vi "Process_data.vi"(0 "PWA Binary":i16[][](array[numeric]), 1 "Analogue Binary":i16[][](array[numeric]), 2 "LDA Binary output":u16[][](array[numeric]), 3 "Analogue volts":dbl[][](array[numeric]) format="%.2f", 4 "Measurement top level?":bool, 5 "Block Timings":T1={"Started"=0.0, "Ended"=0.0, "Analogue Frequency Hz"=1000.0} {"Analogue Frequency Hz" format="%.2f"}) -> (6 "Vel stat display":string[][](table), 7 "First Plot data":cluster{"Xo":dbl, "Delta X":dbl, dbl[]}[](array[cluster]) {"?" format="%.2f"; "Delta X" format="%.2f"; "Xo" format="%.2f"}, 8 "Second Plot data":cluster{"Xo":dbl, "Delta X":dbl, dbl[]}[](array[cluster]) {"?" format="%.2f"; "Delta X" format="%.2f"; "Xo" format="%.2f"}, 9 "Max Measurement time up":bool)   [LabVIEW 2010]
uses:
  Controls/Block_start_and_end.ctl
  Controls/Correlation_cluster.ctl
  Controls/Inst_type.ctl
  Controls/Instrument_Array.ctl
  Controls/Board_Types.ctl
  Globals/Meas_global.vi
  Globals/LDA_meas_global_1.vi
  Acquisition/PWA/PWAtasksGLOBAL.vi
  Globals/Dynamic_call_global.ph.vi
  Globals/Plug_in_data_global.vi
  <vilib>/Analysis/NI_AALBase.lvlib
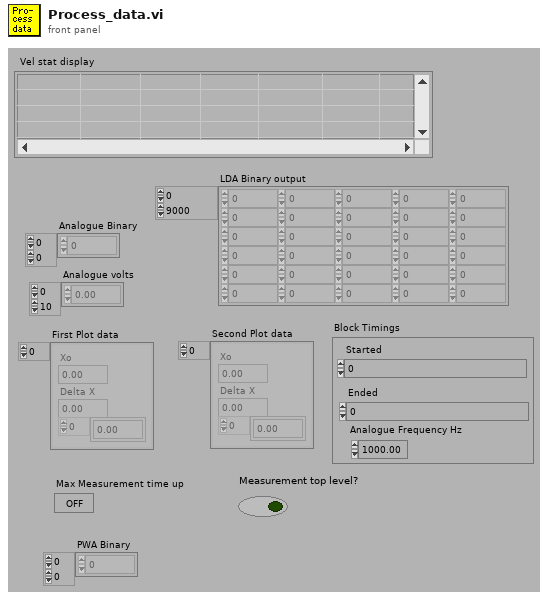
[diagram p1: front panel]
types:
  T1 = typedef "Block_start_and_end.ctl" = cluster{"Started":dbl, "Ended":dbl, "Analogue Frequency Hz":dbl}
  T2 = typedef "PWA_Data.ctl" = enum16{"No PWA Data", "One Ch PWA"}
  T3 = typedef "BSA_Type.ctl" = enum16{"57N11", "BSA F60"}
  T4 = typedef "Correlation_cluster.ctl" = cluster{"U inst":string, "W inst":string, "uw":dbl, "uw/u'w'":dbl, "u^2w":dbl, "uw^2":dbl, "uw^3":dbl, "u^3w":dbl, "u^2w^2":dbl}
  T5 = typedef "Inst_type.ctl" = enum16{"Propeller anemometer", "Raw voltage", "Pressure Transducer", "Pitot-static tube", "Preston tube", "Hot wire", "Cross wire 1", "Cross wire 2", "Generic Linear", "Generic Polynomial", "Generic BackPoly", "Fast FID", "Thermocouple", "Cold wire", "Pulsed Wire", "LDA Vel", "LDA Tran time", "LDA Arr time"}
  T6 = typedef "Instrument_Array.ctl" = enum16{"PWA", "LDA", "Analogue"}
  T7 = typedef "Board_Types.ctl" = enum16{"Simulate", "NB-MIO-16H", "PCI-MIO-16E", "6000E Series", "USB-92xx", "ADC488", "Lab-NB", "NB-DIO-24", "NI-DAQmx", "Local ADAM", "Server Channels"}
  T8 = typedef "Analysis_info_cluster.ctl" = cluster{"Colour":u32, "Inst type":T5, "Inst name":string, "Symbol":string, "Code name":string, "Extra Info":string, "Inst Array":T6, "Index":i32, "Voltage Index":i32, "Extra Titles":string[], "Extra Values":string[]}
  T9 = typedef "Post_Process.ctl" = enum16{"Take New Data", "Post Process Raw Data File"}
  T10 = typedef "Graph_Type.ctl" = enum16{"Show no graph", "Voltage trace", "Velocity trace", "Vel histogram", "Spectrum", "f.E(f) v Log f", "Auto-Corr"}
  T11 = cluster{"Plot 1":u16, "Plot 2":u16, "Save graph":u16, "Plot Type":T10}
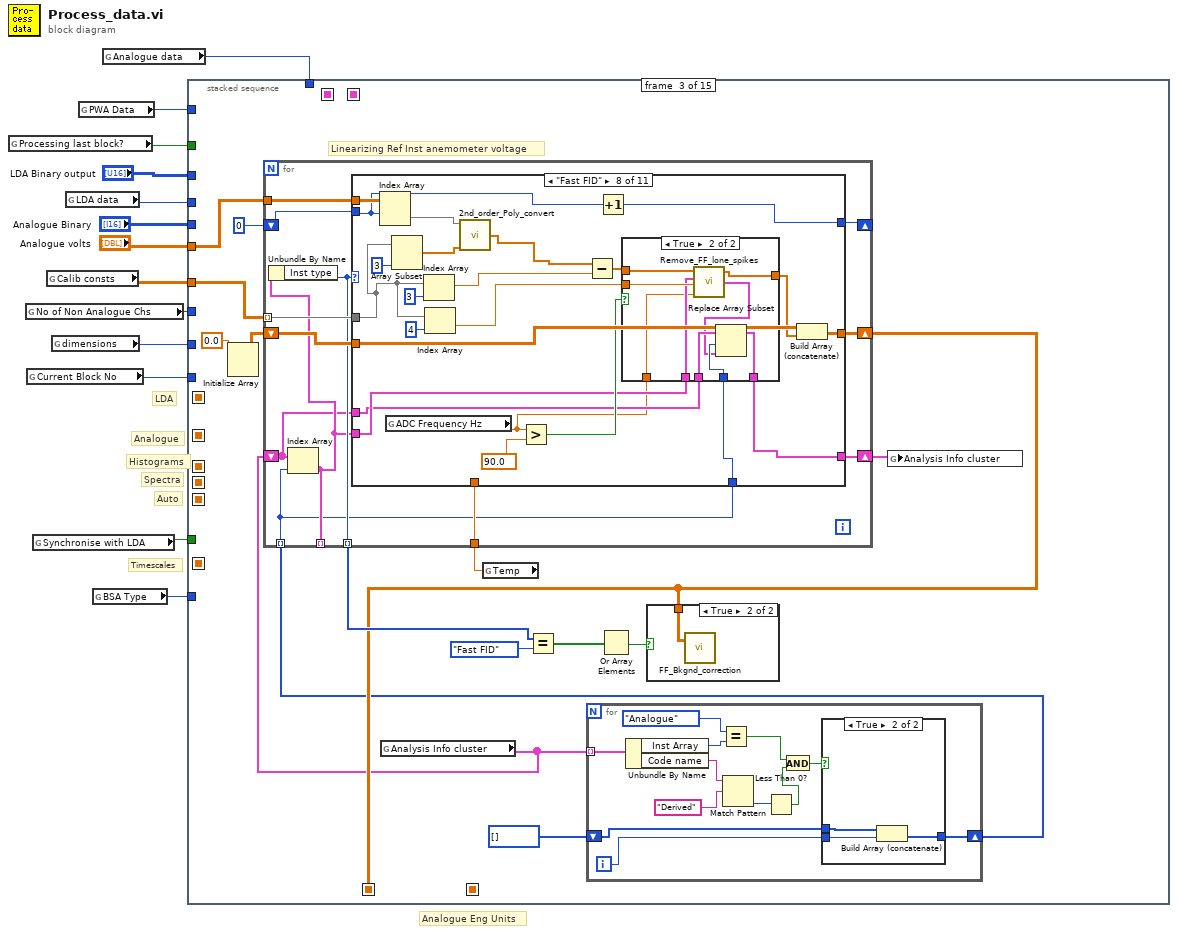
[diagram p0: block diagram]
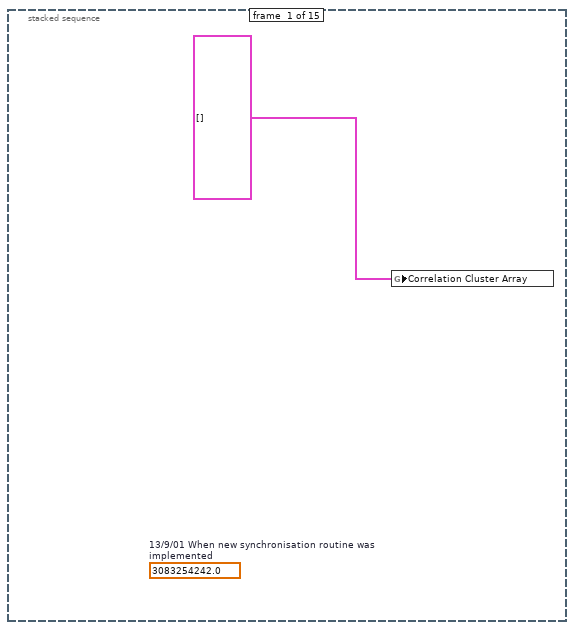
[diagram p2: hidden frame]
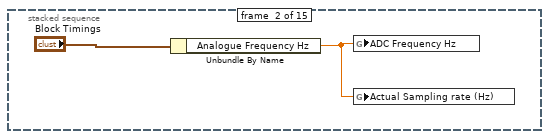
[diagram p3: hidden frame]
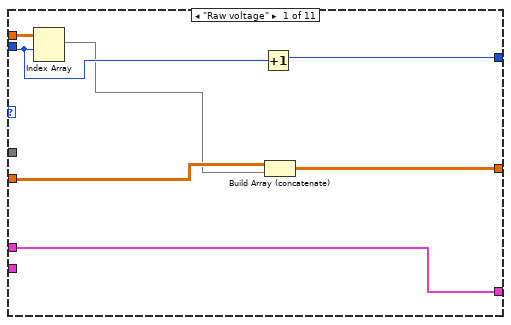
[diagram p6: hidden frame]
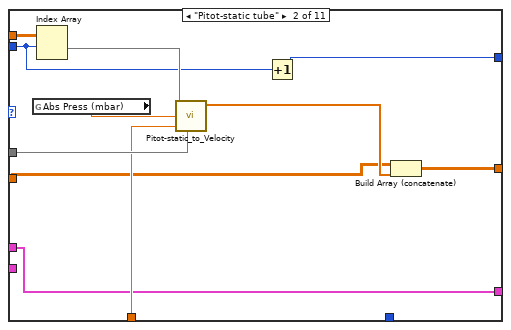
[diagram p7: hidden frame]
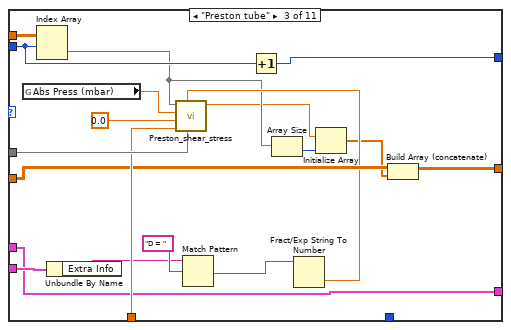
[diagram p8: hidden frame]
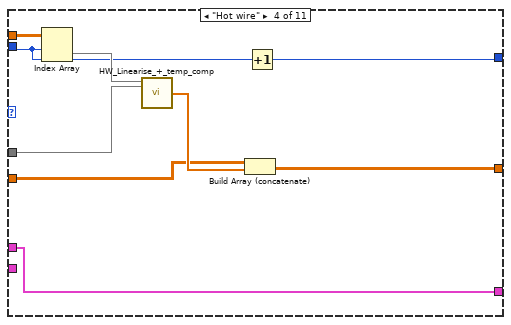
[diagram p9: hidden frame]
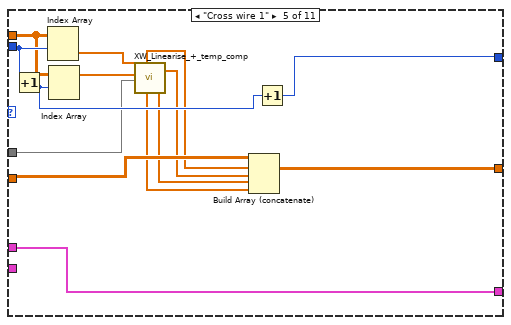
[diagram p10: hidden frame]
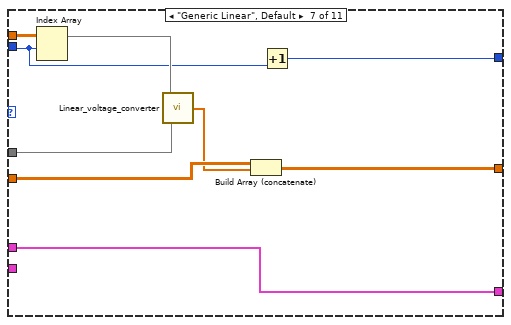
[diagram p12: hidden frame]
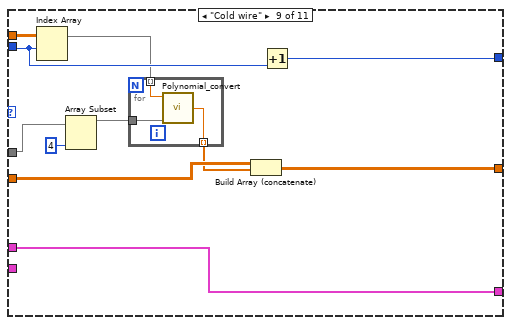
[diagram p14: hidden frame]
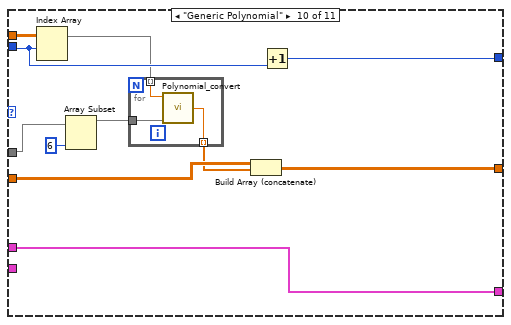
[diagram p15: hidden frame]
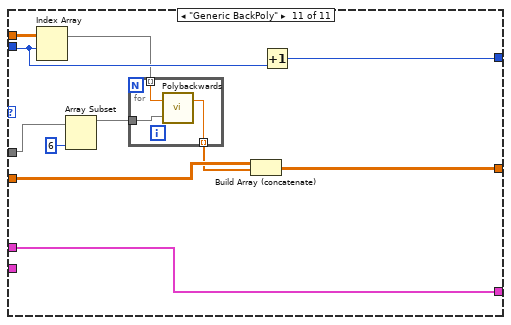
[diagram p16: hidden frame]
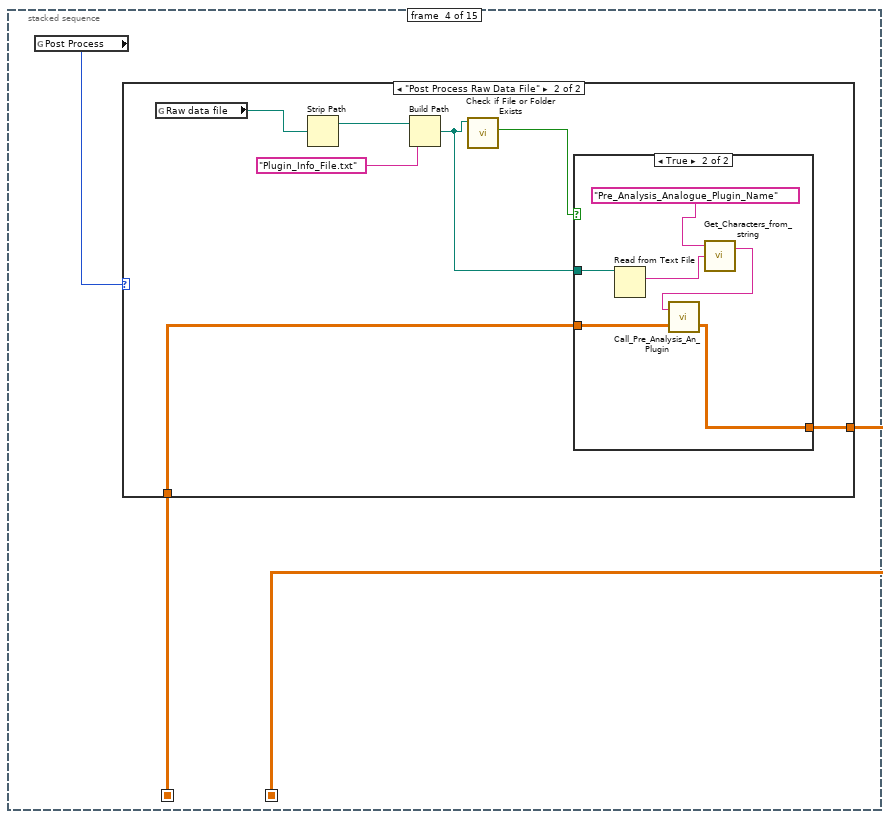
[diagram p17: hidden frame]
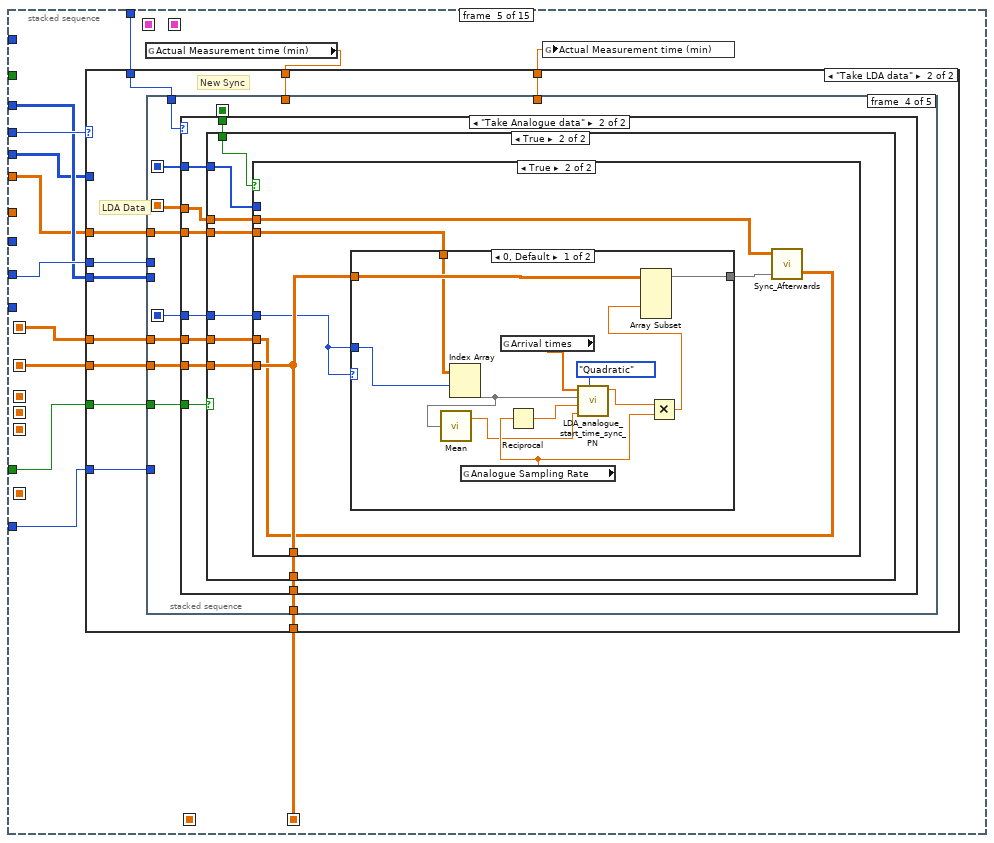
[diagram p20: hidden frame]
diagram:
  # "Timescales"
  # "LDA"
  # "Auto"
  # "Spectra"
  # "Histograms"
  # "Analogue Eng Units"
  # "Analogue"
  n1 = global read "Meas_global.vi" "Processing last block?"() -> (w9:bool)
  n2 = global read "Meas_global.vi" "No of Non Analogue Chs"() -> (w5:i32)
  n3 = global read "Meas_global.vi" "Current Block No"() -> (w10:i32)
  n4 = global read "Meas_global.vi" "Synchronise with LDA"() -> (w4:bool)
  n5 = global read "Meas_global.vi" "Calib consts"() -> (w3:dbl[][])
  n6 = global read "Meas_global.vi" "dimensions"() -> (w13:enum16{"1D", "2D"})
  n7 = global read "Meas_global.vi" "LDA data"() -> (w12:enum16{"No LDA data", "Take LDA data"})
  n8 = global read "Meas_global.vi" "PWA Data"() -> (w2:T2)
  n9 = global read "LDA_meas_global_1.vi" "BSA Type"() -> (w1:T3)
  n10 = global read "Meas_global.vi" "Analogue data"() -> (w11:enum16{"No Analogue data", "Take Analogue data"})
  n11 = stacked-sequence {
    seq-local: [_ _ _ _ w235 _ _ _ _ _ _ _ _ _ _] -> [_ _ _ _ _ _ w488 w501 w509 w524 w535 w554 w559 _ _]
    seq-local: [_ _ _ w210 _ _ _ _ _ _ _ _ _ _ _] -> [_ _ _ _ w237 _ _ _ _ _ _ _ _ _ _]
    seq-local: [_ _ _ _ _ _ w487 _ _ _ _ _ _ _ _] -> [_ _ _ _ _ _ _ _ _ w523 _ _ _ w602 _]
    seq-local: [_ _ _ _ _ _ _ w500 _ _ _ _ _ _ _] -> [_ _ _ _ _ _ _ _ _ w522 _ _ _ _ _]
    seq-local: [_ _ _ _ _ _ _ _ w508 _ _ _ _ _ _] -> [_ _ _ _ _ _ _ _ _ w521 w542 _ _ _ _]
    seq-local: [_ _ _ _ _ _ _ _ _ w516 _ _ _ _ _] -> [_ _ _ _ _ _ _ _ _ _ _ _ w565 _ _]
    seq-local: [_ _ _ _ _ _ _ _ _ w515 _ _ _ _ _] -> [_ _ _ _ _ _ _ _ _ _ _ _ w564 _ _]
    seq-local: [_ _ _ _ w232 _ _ _ _ _ _ _ _ _ _] -> [_ _ _ _ _ _ w489 _ _ w514 _ w555 w560 _ w611]
    seq-local: [_ _ _ _ _ _ _ _ _ _ w528 _ _ _ _] -> [_ _ _ _ _ _ _ _ _ _ _ w552 _ _ w610]
    seq-local: [_ _ w21 _ _ _ _ _ _ _ _ _ _ _ _] -> [_ _ _ w209 _ _ _ _ _ _ _ _ _ _ _]
    tunnel: w10 -> [_ _ _ _ _ w387 _ _ _ _ _ _ _ _ _]
    tunnel: w13 -> [_ _ _ _ w239 _ _ _ _ _ _ _ _ _ _]
    tunnel: w12 -> [_ _ _ _ w238 _ _ _ _ _ _ _ _ _ _]
    tunnel: w11 -> [_ _ _ _ w236 _ _ _ _ _ _ _ _ _ _]
    tunnel: w9 -> [_ _ _ _ _ _ _ _ _ _ _ _ _ w603 _]
    tunnel: "LDA Binary output" -> [_ _ _ _ w234 _ _ _ _ _ _ _ w563 _ _]
    tunnel: "Analogue Binary" -> [_ _ _ _ w229 _ _ _ _ _ _ _ w562 w601 _]
    tunnel: "Analogue volts" -> [_ _ w27 _ w228 _ _ _ _ w513 _ _ w561 w596 _]
    tunnel: w5 -> [_ _ _ _ _ _ _ _ _ _ _ _ _ _ _]
    tunnel: w4 -> [_ _ _ _ w233 _ _ _ _ _ _ _ _ _ _]
    tunnel: w3 -> [_ _ w26 _ _ _ _ _ _ _ _ _ _ _ _]
    tunnel: w2 -> [_ _ _ _ _ w391 _ _ _ _ _ _ _ _ _]
    tunnel: w1 -> [_ _ _ _ w227 _ _ _ _ _ _ _ _ _ _]
    frame #0 {
      (unwired) 3083254242.0  # 13/9/01 When new synchronisation routine was implemented
      n12 = global write "Meas_global.vi" "Correlation Cluster Array"(T4[] [] ("Correlation Cluster Array")) -> ()
    }
    frame #1 {
      n13 = Unbundle By Name("Block Timings") -> ("Analogue Frequency Hz"=w15:dbl)
      n14 = global write "LDA_meas_global_1.vi" "ADC Frequency Hz"(w15) -> ()
      n15 = global write "Meas_global.vi" "Actual Sampling rate (Hz)"(w15) -> ()
    }
    frame #2 {
      # "Linearizing Ref Inst anemometer voltage"
      n16 = Initialize Array(0.0) -> (w29:dbl[][])  [unwired: 2 out]
      n17 = global read "Meas_global.vi" "Analysis Info cluster"() -> (w18:T8[])
      n18 = global read "Meas_global.vi" "Temp"() -> (w28:dbl)
      n19 = for {
        tunnel: w18 -> [w35] mode=indexing
        shift-right: [w32] -> w17
        shift-left: i32[] [] -> [w33]
        i -> [w34]
        n20 = Unbundle By Name(w35) -> ("Inst Array"=w43:T6, "Code name"=w41:string)
        n21 = Equal?(x=Instrument_Array."Analogue" ("Inst Array"), y=w43) -> (x = y?=w37:bool)
        n22 = Match Pattern(string=w41, regular expression="Derived") -> (offset past match=w39:i32)  [unwired: 4 out]
        n23 = Less Than 0?(x=w39) -> (x < 0?=w38:bool)
        n24 = And(x=w37, y=w38) -> (x .and. y?=w36:bool)
        n25 = case shown="True" w36 {
          tunnel: w34 -> [_ w47]
          tunnel: w33 -> [w44 w46]
          tunnel: [w44 w45] -> w32
          frame False {
          }
          frame True {
            n26 = Build Array (concatenate)(w46, w47) -> (w45:i32[])
          }
        }
      }
      n27 = for {
        tunnel: w27 -> [w56]
        tunnel: w26 -> [w60] mode=indexing
        shift-right: [w59] -> _
        shift-left: 0 -> [w55]
        shift-right: [w57] -> w21
        shift-left: w29 -> [w58]
        tunnel: [w52] -> _ mode=indexing
        tunnel: w28 -> [w54]
        tunnel: [w53] -> w24 mode=indexing
        tunnel: w17 -> [w49] mode=indexing
        shift-right: [w50] -> w20
        shift-left: w18 -> [w51]
        n28 = Index Array(array=w51, index=w49) -> (element=w52:T8)
        n29 = Unbundle By Name(w52) -> ("Inst type"=w53:T5)
        n30 = case shown="\"Fast FID\"" w53 {
          tunnel: w60 -> [_ w78 w97 w106 w112 _ w132 w145 w170 w184 w198]
          tunnel: w54 -> [_ w77 w96 _ _ _ _ _ _ _ _]
          tunnel: w55 -> [w65 w74 w94 w103 w120 w122 w129 w144 w176 w190 w204]
          tunnel: w56 -> [w67 w76 w95 w105 w119 _ w131 w155 w177 w191 w205]
          tunnel: [w66 w73 w93 w102 w117 w122 w128 w147 w175 w189 w203] -> w59
          tunnel: w58 -> [w64 w71 w92 w99 w116 w123 w126 w154 w173 w187 w201]
          tunnel: [w63 w70 w91 w100 w115 w123 w127 w137 w174 w188 w202] -> w57
          tunnel: w52 -> [_ _ w87 _ _ _ _ w138 _ _ _]
          tunnel: w51 -> [w61 w68 w79 w98 w107 w121 w124 w135 w167 w181 w195]
          tunnel: [w61 w68 w79 w98 w107 w121 w124 w136 w167 w181 w195] -> w50
          tunnel: w49 -> [_ _ _ _ _ _ _ w134 _ _ _]
          frame "Raw voltage" {
            n31 = Index Array(array=w67, index (row)=w65) -> (element=w62:dbl[])  [unwired: 1 in]
            n32 = Increment(x=w65) -> (x+1=w66:i32)
            n33 = Build Array (concatenate)(w64, w62) -> (w63:dbl[][])
          }
          frame "Pitot-static tube" {
            n34 = global read "Meas_global.vi" "Abs Press (mbar)"() -> (w69:dbl)
            n35 = Index Array(array=w76, index (row)=w74) -> (element=w75:dbl[])  [unwired: 1 in]
            n36 = call "Pitot-static_to_Velocity.vi"("Pressure Trans voltage"=w75, "Atmos Press mbar  (1000)"=w69, "Temp  C  (20)"=w77, "Pressure Trans Calib const"=w78) -> ("Velocity (m/s)"=w72:dbl[])  [unwired: 1 in, 3 out]
            n37 = Increment(x=w74) -> (x+1=w73:i32)
            n38 = Build Array (concatenate)(w71, w72) -> (w70:dbl[][])
          }
          frame "Preston tube" {
            n39 = global read "Meas_global.vi" "Abs Press (mbar)"() -> (w90:dbl)
            n40 = Index Array(array=w95, index (row)=w94) -> (element=w82:dbl[])  [unwired: 1 in]
            n41 = Unbundle By Name(w87) -> ("Extra Info"=w86:string)
            n42 = Match Pattern(string=w86, regular expression="D = " ("String to match")) -> (after substring=w88:string)  [unwired: 4 out]
            n43 = Increment(x=w94) -> (x+1=w93:i32)
            n44 = Array Size(array=w82) -> (size(s)=w83:i32)
            n45 = Fract/Exp String To Number(string=w88) -> (number=w85:dbl)  [unwired: 4 out]
            n46 = call "Preston_shear_stress.vi"("Calib. consts"=w97, "Diam. (mm)"=w85, "Temp (C)"=w96, "Static gauge head mm H2O"=0.0 ("Static gauge press mm H2O"), "Atmos. pressure (mbars)"=w90, "Pressure transducer voltages"=w82) -> ("Mean shear stress (Pa)"=w81:dbl)  [unwired: 1 in, 3 out]
            n47 = Initialize Array(w81, w83) -> (w80:dbl[])
            n48 = Build Array (concatenate)(w92, w80) -> (w91:dbl[][])
          }
          frame "Hot wire" {
            n49 = Index Array(array=w105, index (row)=w103) -> (element=w104:dbl[])  [unwired: 1 in]
            n50 = call "HW_Linearise_+_temp_comp.vi"("Caib const"=w106, "HW voltage"=w104) -> ("Velocity"=w101:dbl[])  [unwired: 3 in, 1 out]
            n51 = Build Array (concatenate)(w99, w101) -> (w100:dbl[][])
            n52 = Increment(x=w103) -> (x+1=w102:i32)
          }
          frame "Cross wire 1" {
            n53 = Increment(x=w120) -> (x+1=w118:i32)
            n54 = Index Array(array=w119, index (row)=w120) -> (element=w114:dbl[])  [unwired: 1 in]
            n55 = Index Array(array=w119, index (row)=w118) -> (element=w113:dbl[])  [unwired: 1 in]
            n56 = call "XW_Linearise_+_temp_comp.vi"("Calib const"=w112, "XW2 voltage"=w113, "XW1 voltage"=w114) -> ("U1"=w109:dbl[], "V"=w111:dbl[], "U2"=w108:dbl[], "U"=w110:dbl[])  [unwired: 1 in]
            n57 = Build Array (concatenate)(w116, w110, w111, w109, w108) -> (w115:dbl[][])
            n58 = Increment(x=w118) -> (x+1=w117:i32)
          }
          frame "Cross wire 2" {
          }
          frame "Generic Linear", Default {
            n59 = Index Array(array=w131, index (row)=w129) -> (element=w130:dbl[])  [unwired: 1 in]
            n60 = call "Linear_voltage_converter.vi"("Caib const A,B"=w132, "Voltage array"=w130) -> ("Converted array"=w125:dbl[])
            n61 = Build Array (concatenate)(w126, w125) -> (w127:dbl[][])
            n62 = Increment(x=w129) -> (x+1=w128:i32)
          }
          frame "Fast FID" {
            n63 = Index Array(array=w155, index (row)=w144) -> (element=w142:dbl[])  [unwired: 1 in]
            n64 = global read "LDA_meas_global_1.vi" "ADC Frequency Hz"() -> (w133:dbl)
            n65 = Array Subset(array=w145, length=3) -> (w143:dbl[])  [unwired: 1 in]
            n66 = Index Array(array=w145, index=3) -> (element=w152:dbl)
            n67 = Index Array(array=w145, index=4) -> (element=w148:dbl)
            n68 = call "2nd_order_Poly_convert.vi"("Calib constants"=w143, "Voltage"=w142) -> ("Eng Values"=w141:dbl[])  [unwired: 4 out]
            n69 = Greater?(x=w133, y=90.0) -> (0:w140:bool)
            n70 = Subtract(x=w141, y=w152) -> (x-y=w151:dbl[])
            n71 = Increment(x=w144) -> (x+1=w147:i32)
            n72 = case shown="True" w140 {
              tunnel: w151 -> [w157 w166]
              tunnel: [w157 w165] -> w139
              tunnel: w148 -> [_ w164]
              tunnel: w138 -> [_ w163]
              tunnel: [w156 w162] -> w136
              tunnel: w135 -> [w156 w161]
              tunnel: w134 -> [_ w160]
              tunnel: w133 -> [_ w158]
              frame False {
              }
              frame True {
                n73 = call "Remove_FF_lone_spikes.vi"("ADC Frequency Hz"=w158, "Bkgnd variance"=w164, "Analysis Info cluster"=w163, "Time Trace"=w166) -> ("Analysis Info cluster out"=w159:T8, "Filtered Time Trace"=w165:dbl[])  [unwired: 1 out]
                n74 = Replace Array Subset(array=w161, new element=w159, index=w160) -> (w162:T8[])
              }
            }
            n75 = Build Array (concatenate)(w154, w139) -> (w137:dbl[][])
          }
          frame "Cold wire" {
            n76 = Index Array(array=w177, index (row)=w176) -> (element=w172:dbl[])  [unwired: 1 in]
            n77 = Array Subset(array=w170, length=4) -> (w169:dbl[])  [unwired: 1 in]
            n78 = for {
              tunnel: w169 -> [w180]
              tunnel: w172 -> [w179] mode=indexing
              tunnel: [w178] -> w171 mode=indexing
              n79 = call "Polynomial_convert.vi"("Calib constants"=w180, "Voltage"=w179) -> ("Eng Values"=w178:dbl)  [unwired: 4 out]
            }
            n80 = Build Array (concatenate)(w173, w171) -> (w174:dbl[][])
            n81 = Increment(x=w176) -> (x+1=w175:i32)
          }
          frame "Generic Polynomial" {
            n82 = Index Array(array=w191, index (row)=w190) -> (element=w186:dbl[])  [unwired: 1 in]
            n83 = Array Subset(array=w184, length=6) -> (w183:dbl[])  [unwired: 1 in]
            n84 = for {
              tunnel: w183 -> [w194]
              tunnel: w186 -> [w193] mode=indexing
              tunnel: [w192] -> w185 mode=indexing
              n85 = call "Polynomial_convert.vi"("Calib constants"=w194, "Voltage"=w193) -> ("Eng Values"=w192:dbl)  [unwired: 4 out]
            }
            n86 = Build Array (concatenate)(w187, w185) -> (w188:dbl[][])
            n87 = Increment(x=w190) -> (x+1=w189:i32)
          }
          frame "Generic BackPoly" {
            n88 = Index Array(array=w205, index (row)=w204) -> (element=w200:dbl[])  [unwired: 1 in]
            n89 = Array Subset(array=w198, length=6) -> (w197:dbl[])  [unwired: 1 in]
            n90 = for {
              tunnel: w197 -> [w208]
              tunnel: w200 -> [w207] mode=indexing
              tunnel: [w206] -> w199 mode=indexing
              n91 = call "Polybackwards.vi"("Coefficients"=w208, "Y input"=w207) -> ("X output"=w206:dbl)  [unwired: 1 out]
            }
            n92 = Build Array (concatenate)(w201, w199) -> (w202:dbl[][])
            n93 = Increment(x=w204) -> (x+1=w203:i32)
          }
        }
      }
      n94 = Equal?(x=w24, y=Inst_type."Fast FID" ("Inst type")) -> (x = y?=w23:bool[])
      n95 = Or Array Elements(Boolean array=w23) -> (logical OR=w22:bool)
      n96 = case shown="True" w22 {
        tunnel: w21 -> [_ w48]
        frame False {
        }
        frame True {
          n97 = call "FF_Bkgnd_correction.vi"("Analogue Data"=w48) -> ()  [unwired: 3 out]
        }
      }
      n98 = global write "Meas_global.vi" "Analysis Info cluster"(w20) -> ()
    }
    frame #3 {
      n99 = global read "Meas_global.vi" "Post Process"() -> (w211:T9)
      n100 = case shown="\"Post Process Raw Data File\"" w211 {
        tunnel: [w212 w218] -> w210
        tunnel: w209 -> [w212 w219]
        frame "Take New Data" {
        }
        frame "Post Process Raw Data File" {
          n101 = global read "Meas_global.vi" "Raw data file"() -> (w217:path)
          n102 = Strip Path(path=w217) -> (stripped path=w216:path)  [unwired: 1 out]
          n103 = Build Path(base path=w216, name or relative path="Plugin_Info_File.txt") -> (appended path=w213:path)
          n104 = call <vilib>:"Check if File or Folder Exists.vi"("path"=w213) -> ("file or folder exists?"=w214:bool)  [unwired: 1 in, 9 out]
          n105 = case shown="True" w214 {
            tunnel: w219 -> [w220 w226]
            tunnel: [w220 w225] -> w218
            tunnel: w213 -> [_ w223]
            frame False {
            }
            frame True {
              n106 = Read from Text File(file (use dialog)=w223) -> (text=w222:string)  [unwired: 1 in, 5 out]
              n107 = call "Get_Characters_from_string.vi"("Input string"=w222, "Variable name"="Pre_Analysis_Analogue_Plugin_Name") -> ("Value"=w221:string)  [unwired: 1 in, 1 out]
              n108 = call "Call_Pre_Analysis_An_Plugin.vi"("Analogue In"=w226, "Plugin Name"=w221) -> ("Analogue Out"=w225:dbl[][])  [unwired: 1 out]
            }
          }
        }
      }
    }
    frame #4 {
      n109 = global read "Meas_global.vi" "Actual Measurement time (min)"() -> (w231:dbl)
      n110 = case shown="\"Take LDA data\"" w238 {
        tunnel: w234 -> [_ w262]
        tunnel: [w251 w256] -> w235
        tunnel: w239 -> [_ w261]
        tunnel: w237 -> [w251 w260]
        tunnel: w236 -> [_ w259]
        tunnel: w233 -> [_ w258]
        tunnel: [dbl[][] [] w257] -> w232
        tunnel: w231 -> [w241 w255]
        tunnel: [w240 w254] -> w230
        tunnel: w229 -> [w247 _]
        tunnel: w228 -> [_ w253]
        tunnel: w227 -> [_ w252]
        frame "No LDA data" {
          n111 = Array Size(array=w247) -> (size(s)=w249:i32[])
          n112 = global read "Meas_global.vi" "Actual Sampling rate (Hz)"() -> (w246:dbl)
          n113 = Index Array(array=w249, index=1) -> (element=w245:i32)
          n114 = Divide(x=w245, y=w246) -> (x/y=w243:dbl)
          n115 = Divide(x=w243, y=60.0) -> (x/y=w242:dbl)
          n116 = Add(x=w241, y=w242) -> (x+y=w240:dbl)
        }
        frame "Take LDA data" {
          # "New Sync"
          # "LDA Data"
          n117 = stacked-sequence {
            seq-local: [_ w277 _ _ _] -> [_ _ _ w324 _]
            seq-local: [w266 _ _ _ _] -> [_ w269 w292 w320 _]
            seq-local: [_ w270 _ _ _] -> [_ _ _ w319 _]
            seq-local: [_ _ w290 _ _] -> [_ _ _ w318 _]
            tunnel: w261 -> [_ w278 _ _ _]
            tunnel: w262 -> [_ w276 _ _ _]
            tunnel: w260 -> [_ _ _ w325 _]
            tunnel: w259 -> [_ _ _ w326 _]
            tunnel: w258 -> [w267 _ _ w323 _]
            tunnel: [_ _ _ w322 _] -> w257
            tunnel: [_ _ _ w321 _] -> w256
            tunnel: w255 -> [_ _ _ _ w380]
            tunnel: [_ _ _ _ w379] -> w254
            tunnel: w253 -> [_ _ _ w317 _]
            tunnel: w252 -> [_ w268 _ _ _]
            frame #0 {
              w264 = 3083254242.0  # 13/9/01 When new synchronisation routine was implemented
              n118 = global read "Meas_global.vi" "Time Data was Aquired"() -> (w265:dbl)
              n119 = Greater?(x=w265, y=w264) -> (0:w263:bool)
              n120 = Compound Arithmetic op=AND(w267, w263) -> (w266:bool)
            }
            frame #1 {
              n121 = Array Size(array=w276) -> (size(s)=w275:i32[])
              n122 = Index Array(array=w275, index=1 ("Index")) -> (element=w273:i32)
              n123 = Greater?(x=w273, y=1) -> (0:w271:bool)
              n124 = case shown="True" w271 {
                tunnel: w276 -> [_ w288]
                tunnel: w278 -> [_ w287]
                tunnel: [w282 w285] -> w277
                tunnel: [i32[] [] ("Sync Index") w286] -> w270
                tunnel: w269 -> [_ w289]
                tunnel: w268 -> [_ _]
                frame False {
                  w280 = 0 ("Dimension Size")
                  n125 = Initialize Array(0.0, w280, w280) -> (w282:dbl[][])
                  n126 = global write "LDA_meas_global_1.vi" "Arrival times"(dbl[] [] ("Weighting array")) -> ()
                }
                frame True {
                  n127 = Not(x=w289) -> (.not. x?=w284:bool)
                  n128 = call "LDA_High_Convert_New.vi"("LDA Binary data"=w288, "dimensions"=w287, "Create Sync Index"=w284) -> ("LDA data"=w285:dbl[][], "Sync Index"=w286:i32[])  [unwired: 2 out]
                }
              }
            }
            frame #2 {
              n129 = global read "Meas_global.vi" "Board type"() -> (w295:T7)
              n130 = Equal?(x=Board_Types."NI-DAQmx" ("Board type"), y=w295) -> (x = y?=w293:bool)
              n131 = And(x=w293, y=w292) -> (x .and. y?=w291:bool)
              n132 = case shown="True" w291 {
                tunnel: [-1 ("f") w298] -> w290
                frame False {
                }
                frame True {
                  n133 = global read "Meas_global.vi" "Analysis Info cluster"() -> (w297:T8[])
                  n134 = Array Size(array=w297) -> (size(s)=w303:i32)
                  n135 = Decrement(x=w303) -> (x-1=w302:i32)
                  n136 = while {
                    tunnel: w297 -> [w316] mode=indexing
                    tunnel: w302 -> [w308]
                    tunnel: [w305] -> w301
                    tunnel: [w304] -> w300
                    i -> [w307]
                    stop <- w309 stop-if-true
                    n137 = Unbundle By Name(w316) -> ("Voltage Index"=w304:i32, "Inst type"=w314:T5, "Symbol"=w312:string)
                    n138 = Equal?(x=w307, y=w308) -> (x = y?=w306:bool)
                    n139 = Equal?(x=Inst_type."Raw voltage" ("Inst type"), y=w314) -> (x = y?=w310:bool)
                    n140 = Equal?(x="Sync", y=w312) -> (x = y?=w311:bool)
                    n141 = And(x=w310, y=w311) -> (x .and. y?=w305:bool)
                    n142 = Or(x=w305, y=w306) -> (x .or. y?=w309:bool)
                  }
                  n143 = Select(t=w300, s=w301, f=-1) -> (s? t:f=w298:i32)
                }
              }
            }
            frame #3 {
              n144 = case shown="\"Take Analogue data\"" w326 {
                tunnel: w325 -> [_ w337]
                tunnel: w324 -> [w328 w336]
                tunnel: w323 -> [_ w335]
                tunnel: [w328 w334] -> w322
                tunnel: [dbl[][] [] w333] -> w321
                tunnel: w320 -> [_ w332]
                tunnel: w319 -> [_ w331]
                tunnel: w318 -> [_ w330]
                tunnel: w317 -> [_ w329]
                frame "No Analogue data" {
                }
                frame "Take Analogue data" {
                  n145 = case shown="True" w335 {
                    tunnel: w337 -> [w339 w344]
                    tunnel: [w338 w343] -> w334
                    tunnel: w336 -> [w338 w347]
                    tunnel: [w339 w342] -> w333
                    tunnel: w332 -> [_ w345]
                    tunnel: w331 -> [_ w346]
                    tunnel: w330 -> [_ w341]
                    tunnel: w329 -> [_ w340]
                    frame False {
                    }
                    frame True {
                      n146 = case shown="True" w345 {
                        tunnel: w347 -> [w353 w365]
                        tunnel: w346 -> [w350 _]
                        tunnel: w344 -> [w349 w364]
                        tunnel: [w352 w361] -> w343
                        tunnel: [dbl[][] [] w364] -> w342
                        tunnel: w341 -> [_ w360]
                        tunnel: w340 -> [_ w362]
                        frame False {
                          n147 = for {
                            tunnel: w350 -> [w356]
                            tunnel: w349 -> [w355] mode=indexing
                            tunnel: [w354] -> w348 mode=indexing
                            n148 = for {
                              tunnel: w356 -> [w359] mode=indexing
                              tunnel: w355 -> [w358]
                              tunnel: [w357] -> w354 mode=indexing
                              n149 = Index Array(array=w358, index=w359) -> (element=w357:dbl)
                            }
                          }
                          n150 = Build Array (concatenate)(w353, w348) -> (w352:dbl[][])
                        }
                        frame True {
                          n151 = case shown="0, Default" w360 {
                            tunnel: w364 -> [w377 w378]
                            tunnel: [w376 w378] -> w363
                            tunnel: w362 -> [w370 _]
                            tunnel: w360 -> [w368 _]
                            frame 0, Default {
                              n152 = Index Array(array=w370, index (row)=w368) -> (element=w367:dbl[])  [unwired: 1 in]
                              n153 = call <vilib>:"Mean.vi"("X"=w367) -> ("mean"=w366:dbl)  [unwired: 1 out]
                              n154 = global read "Meas_global.vi" "Analogue Sampling Rate"() -> (w372:dbl)
                              n155 = global read "LDA_meas_global_1.vi" "Arrival times"() -> (w375:dbl[])
                              n156 = Reciprocal(x=w372) -> (1/x=w374:dbl)
                              n157 = call "LDA_analogue_start_time_sync_PN.vi"("Correlation peak fit method"=enum32{"Max", "Quadratic", "Gaussian"}."Quadratic", "Pulse high threshold (Volts)"=w366, "Analogue dt (s)"=w374, "Analogue LDA burst pulse array"=w367, "LDA arrival dt array"=w375) -> ("LDA start time rel. to Analogue (s)"=w373:dbl)  [unwired: 3 out]
                              n158 = Multiply(x=w373, y=w372) -> (x*y=w369:dbl)
                              n159 = Array Subset(array=w377, index (col)=w369) -> (w376:dbl[][])  [unwired: 3 in]
                            }
                            frame -1 {
                            }
                          }
                          n160 = call "Sync_Afterwards.vi"("Analogue Data"=w363, "LDA Data"=w365) -> ("Eng Values"=w361:dbl[][])  [unwired: 2 out]
                        }
                      }
                    }
                  }
                }
              }
            }
            frame #4 {
              n161 = global read "LDA_meas_global_1.vi" "Time for last Block (s)"() -> (w382:dbl)
              n162 = Divide(x=w382, y=60.0) -> (x/y=w381:dbl)
              n163 = Add(x=w380, y=w381) -> (x+y=w379:dbl)
            }
          }
        }
      }
      n164 = global write "Meas_global.vi" "Actual Measurement time (min)"(w230) -> ()
    }
    frame #5 {
      n165 = case shown="\"One Ch PWA\"" w391 {
        tunnel: "PWA Binary" -> [_ w410]
        tunnel: [w393 w406] -> w389
        tunnel: [w393 w405] -> w388
        tunnel: w387 -> [_ w401]
        tunnel: [w392 w399] -> w385
        tunnel: [w392 w398] -> w386
        tunnel: [w392 w395] -> w384
        frame "No PWA Data" {
          w392 = 0 ("y")
          w393 = dbl[][] []
        }
        frame "One Ch PWA" {
          w396 = 0 ("y")
          n166 = global read "PWAtasksGLOBAL.vi" "Probe Rotated Thro' 180"() -> (w394:bool)
          n167 = global read "PWAtasksGLOBAL.vi" "Minimum TOF Index"() -> (w404:i16)
          n168 = global read "PWAtasksGLOBAL.vi" "PWA Lookup Table"() -> (w403:dbl[])
          n169 = Equal?(x=w401, y=1) -> (x = y?=w397:bool)
          n170 = Index Array(array=w410, index (row)=0) -> (element=w409:i16[])  [unwired: 1 in]
          n171 = global read "PWAtasksGLOBAL.vi" "PWA Seconds per clock pulse"() -> (w402:dbl)
          n172 = for {
            tunnel: w409 -> [w432] mode=indexing
            tunnel: [w434] -> w408 mode=indexing
            tunnel: [w433] -> w407 mode=indexing
            tunnel: w404 -> [w431]
            tunnel: w403 -> [w430]
            tunnel: w402 -> [w429]
            shift-right: [w428] -> w399
            shift-left: _ -> [w426]
            shift-right: [w427] -> w398
            shift-left: _ -> [w425]
            tunnel: w396 -> [w424]
            tunnel: w396 -> [w423]
            tunnel: w397 -> [w420]
            tunnel: w396 -> [w417]
            shift-right: [w413] -> w395
            shift-left: _ -> [w415]
            tunnel: w394 -> [w412]
            i -> [w422]
            n173 = Equal To 0?(x=w422) -> (x = 0?=w421:bool)
            n174 = And(x=w420, y=w421) -> (x .and. y?=w416:bool)
            n175 = Select(t=w424, s=w416, f=w426) -> (s? t:f=w419:i32)
            n176 = Select(t=w423, s=w416, f=w425) -> (s? t:f=w418:i32)
            n177 = Select(t=w417, s=w416, f=w415) -> (s? t:f=w414:i32)
            n178 = case shown="-4095" w432 {
              tunnel: w432 -> [w443 _ _]
              tunnel: [w448 w481 w486] -> w434
              tunnel: [w449 w481 w486] -> w433
              tunnel: w431 -> [w447 _ _]
              tunnel: w430 -> [w445 _ _]
              tunnel: w429 -> [w442 _ _]
              tunnel: w419 -> [w441 w480 w485]
              tunnel: [w440 w479 w484] -> w428
              tunnel: [w438 w478 w483] -> w427
              tunnel: w418 -> [w439 w478 w483]
              tunnel: w414 -> [w437 w477 w482]
              tunnel: [w436 w477 w482] -> w413
              tunnel: w412 -> [w435 _ _]
              frame 0, Default {
                n179 = Absolute Value(x=w443) -> (abs(x)=w444:i16)
                n180 = Greater?(x=w444, y=w447) -> (0:w446:bool)
                n181 = case shown="True" w446 {
                  tunnel: [w454 w470] -> w449
                  tunnel: [w454 w458] -> w448
                  tunnel: w443 -> [_ w469]
                  tunnel: w445 -> [_ w466]
                  tunnel: w442 -> [_ w464]
                  tunnel: w441 -> [w453 w462]
                  tunnel: [w453 w462] -> w440
                  tunnel: w439 -> [w452 w461]
                  tunnel: [w451 w461] -> w438
                  tunnel: w437 -> [w450 w455]
                  tunnel: [w450 w456] -> w436
                  tunnel: w435 -> [_ w460]
                  frame False {
                    w454 = nan
                    n182 = Increment(x=w452) -> (x+1=w451:i32)
                  }
                  frame True {
                    n183 = To Double Precision Float(number=w469) -> (double precision float=w465:dbl)
                    n184 = Add(x=w469, y=i16 4095) -> (x+y=w467:i16)
                    n185 = Multiply(x=w464, y=w465) -> (x*y=w463:dbl)
                    n186 = Index Array(array=w466, index=w467) -> (element=w459:dbl)
                    n187 = Reciprocal(x=w463) -> (1/x=w470:dbl)
                    n188 = case shown="False" w460 {
                      tunnel: w459 -> [w474 w476]
                      tunnel: [w474 w475] -> w458
                      frame False {
                      }
                      frame True {
                        n189 = Negate(x=w476) -> (-x=w475:dbl)
                      }
                    }
                    n190 = Less Than 0?(x=w458) -> (x < 0?=w457:bool)
                    n191 = case shown="False" w457 {
                      tunnel: [w471 w473] -> w456
                      tunnel: w455 -> [w471 w472]
                      frame False {
                      }
                      frame True {
                        n192 = Increment(x=w472) -> (x+1=w473:i32)
                      }
                    }
                  }
                }
              }
              frame 4095 {
                w481 = 0.0 ("Eng Values")
                n193 = Increment(x=w480) -> (x+1=w479:i32)
              }
              frame -4095 {
                w486 = 0.0 ("Eng Values")
                n194 = Increment(x=w485) -> (x+1=w484:i32)
              }
            }
          }
          n195 = Build Array(w407) -> (w406:dbl[][])
          n196 = Build Array(w408) -> (w405:dbl[][])
        }
      }
      n197 = global write "PWAtasksGLOBAL.vi" "PWA No of Reverse samples"(w384) -> ()
      n198 = global write "PWAtasksGLOBAL.vi" "PWA No of  TOF Below Min"(w386) -> ()
      n199 = global write "PWAtasksGLOBAL.vi" "PWA No of  TOF Timeouts"(w385) -> ()
      n200 = global write "PWAtasksGLOBAL.vi" "PWA 1/TOF"(w389) -> ()
      n201 = global write "PWAtasksGLOBAL.vi" "PWA Data"(w388) -> ()
    }
    frame #6 {
      n202 = global read "Meas_global.vi" "Histogram control"() -> (w492:i32[])
      n203 = Array Size(array=w492) -> (size(s)=w491:i32)
      n204 = Greater Than 0?(x=w491) -> (x > 0?=w490:bool)
      n205 = case shown="True" w490 {
        tunnel: w489 -> [_ w496]
        tunnel: w488 -> [_ w495]
        tunnel: [w493 w494] -> w487
        frame False {
          w493 = dbl[][] []  # DBL 2D array
        }
        frame True {
          n206 = call "Multi_Histogram.vi"("Equi Spaced"=w495, "Vari Spaced"=w496) -> ("Histogram"=w494:dbl[][])  [unwired: 5 out]
        }
      }
    }
    frame #7 {
      n207 = global read "Meas_global.vi" "Spectra control"() -> (w498:i32[])
      n208 = Array Size(array=w498) -> (size(s)=w499:i32)
      n209 = Greater Than 0?(x=w499) -> (x > 0?=w497:bool)
      n210 = case shown="True" w497 {
        tunnel: w501 -> [_ w504]
        tunnel: [w502 w503] -> w500
        frame False {
          w502 = dbl[][] []  # DBL 2D array
        }
        frame True {
          n211 = call "Multi_spectra.vi"("Equi Spaced"=w504) -> ("Spectra"=w503:dbl[][])  [unwired: 6 out]
        }
      }
    }
    frame #8 {
      n212 = global read "Meas_global.vi" "Auto-Corr control"() -> (w506:i32[])
      n213 = Array Size(array=w506) -> (size(s)=w507:i32)
      n214 = Greater Than 0?(x=w507) -> (x > 0?=w505:bool)
      n215 = case shown="True" w505 {
        tunnel: w509 -> [_ w512]
        tunnel: [w510 w511] -> w508
        frame False {
          w510 = dbl[][] []  # DBL 2D array
        }
        frame True {
          n216 = call "Multi_Auto-Correlation.vi"("Velocity arrays"=w512) -> ("Auto-Corr"=w511:dbl[][])  [unwired: 6 out]
        }
      }
    }
    frame #9 {
      w517 = 2  # Plot No
      w518 = 1  # Plot No
      n217 = global read "Meas_global.vi" "First Graph"() -> (w519:T11)
      n218 = call "Plotter_data.vi"("Vari Spaced"=w514, "Plot No"=w518, "Voltages"=w513, "Equi Spaced"=w524, "Histogram"=w523, "Spectra"=w522, "Auto-correlation"=w521, "Graph"=w519) -> ("Plot data"=w516:cluster{"Xo":dbl, "Delta X":dbl, dbl[]}[])  [unwired: 7 out]
      "First Plot data" <- w516
      n219 = global read "Meas_global.vi" "Second Graph"() -> (w520:T11)
      n220 = call "Plotter_data.vi"("Vari Spaced"=w514, "Plot No"=w517, "Voltages"=w513, "Equi Spaced"=w524, "Histogram"=w523, "Spectra"=w522, "Auto-correlation"=w521, "Graph"=w520) -> ("Plot data"=w515:cluster{"Xo":dbl, "Delta X":dbl, dbl[]}[])  [unwired: 7 out]
      "Second Plot data" <- w515
    }
    frame #10 {
      n221 = global read "Meas_global.vi" "No of Non Analogue Chs"() -> (w525:i32)
      n222 = Array Size(array=w535) -> (size(s)=w536:i32[])
      n223 = Index Array(array=w536, index=0) -> (element=w527:i32)
      n224 = global read "LDA_meas_global_1.vi" "LDA Timescales"() -> (w533:dbl[])
      n225 = global read "PWAtasksGLOBAL.vi" "PWA Timescales"() -> (w532:dbl[])
      n226 = Add(x=w525, y=w527) -> (x+y=w526:i32)
      n227 = Initialize Array(nan, w526) -> (w531:dbl[])
      n228 = Build Array (concatenate)(w533, w532, w531) -> (w530:dbl[])
      n229 = Array Size(array=w542) -> (size(s)=w541:i32[])
      n230 = Index Array(array=w541, index=1) -> (element=w538:i32)
      n231 = global read "Meas_global.vi" "Analogue Sampling Rate"() -> (w539:dbl)
      n232 = global read "Meas_global.vi" "Auto-Corr control"() -> (w529:i32[])
      n233 = for {
        tunnel: w542 -> [w550] mode=indexing
        tunnel: w538 -> [w551]
        tunnel: w539 -> [w549]
        shift-right: [w548] -> w528
        shift-left: w530 -> [w547]
        tunnel: w529 -> [w545] mode=indexing
        tunnel: w525 -> [w544]
        n234 = call "Calculate_Timescales.vi"("Sampling Frequency (Hz)"=w549, "Autocorrelation length"=w551, "Autocorrelation"=w550) -> ("Time Scale estimate (s)"=w546:dbl)
        n235 = Add(x=w545, y=w544) -> (x+y=w543:i32)
        n236 = Replace Array Subset(array=w547, new element=w546, index=w543) -> (w548:dbl[])
      }
      n237 = global write "Meas_global.vi" "Timescales (s)"(w528) -> ()
    }
    frame #11 {
      n238 = call "All_stats.vi"("Timescales"=w552, "Equi Spaced"=w554, "LDA"=w555) -> ("Stats array"=w553:string[])  [unwired: 2 out]
      n239 = global write "Meas_global.vi" "Vel stats info for files"(w553) -> ()
    }
    frame #12 {
      n240 = global read "Dynamic_call_global.ph.vi" "Per Block Plug Ins"() -> (w558:string[])
      n241 = global read "Dynamic_call_global.ph.vi" "Per Block Plug Ins Extra"() -> (w557:string[])
      n242 = Build Array (concatenate)(w558, w557) -> (w556:string[])
      n243 = stacked-sequence {
        seq-local: [w566 _] -> [_ w593]
        tunnel: w560 -> [w579 _]
        tunnel: w561 -> [w578 _]
        tunnel: w563 -> [w574 _]
        tunnel: w562 -> [w575 _]
        tunnel: w565 -> [w571 _]
        tunnel: w564 -> [w569 _]
        tunnel: w559 -> [w568 _]
        tunnel: w556 -> [w567 w592]
        frame #0 {
          n244 = global write "Plug_in_data_global.vi" "Equi Spaced"(w568) -> ()
          n245 = Array Size(array=w567) -> (size(s)=w581:i32)
          n246 = Greater Than 0?(x=w581) -> (x > 0?=w566:bool)
          n247 = case shown="True" w566 {
            tunnel: [w582 w591] -> w580
            tunnel: w579 -> [_ w591]
            tunnel: w578 -> [_ w590]
            tunnel: [w582 w590] -> w577
            tunnel: [i16[][] [] ("Analogue Binary") w589] -> w576
            tunnel: w575 -> [_ w589]
            tunnel: w574 -> [_ w588]
            tunnel: [u16[][] [] ("LDA Binary output") w588] -> w573
            tunnel: [w583 w587] -> w572
            tunnel: w571 -> [_ w587]
            tunnel: [w583 w586] -> w570
            tunnel: w569 -> [_ w586]
            frame False {
              w583 = cluster{"Xo":dbl, "Delta X":dbl, dbl[]}[] [] ("Plot data")
              w582 = dbl[][] [] ("Filtered data")
            }
            frame True {
            }
          }
          n248 = global write "Plug_in_data_global.vi" "Second Plot data"(w570) -> ()
          n249 = global write "Plug_in_data_global.vi" "Analogue Binary"(w576) -> ()
          n250 = global write "Plug_in_data_global.vi" "First Plot data"(w572) -> ()
          n251 = global write "Plug_in_data_global.vi" "LDA Binary"(w573) -> ()
          n252 = global write "Plug_in_data_global.vi" "Vari Spaced"(w580) -> ()
          n253 = global write "Plug_in_data_global.vi" "Voltages"(w577) -> ()
        }
        frame #1 {
          n254 = case shown="True" w593 {
            tunnel: w592 -> [_ w595]
            frame False {
            }
            frame True {
              n255 = call "Analyse_string_array.vi"("String array"=w595) -> ("Unique strings"=w594:string[])  [unwired: 2 out]
              n256 = call "Call_Block_plug_ins.vi"("Per Block Plug Ins"=w594) -> ()
            }
          }
        }
      }
    }
    frame #13 {
      n257 = global read "Meas_global.vi" "Board type"() -> (w597:T7)
      n258 = case shown="\"NI-DAQmx\"" w597 {
        tunnel: w601 -> [w605 _]
        tunnel: [w604 w607] -> w600
        tunnel: w596 -> [_ w606]
        frame "Simulate", Default {
          n259 = call "Analogue_overflow_checker.vi"("I16 data"=w605) -> ("Over/Under string"=w604:string)  [unwired: 2 out]
        }
        frame "NI-DAQmx" {
          n260 = call "Voltage_overflow_checker.vi"("Voltages"=w606) -> ("Over/Under string"=w607:string)  [unwired: 2 out]
        }
      }
      n261 = Empty String/Path?(string/path=w600) -> (empty?=w599:bool)
      n262 = And(x=w603, y=w599) -> (x .and. y?=w598:bool)
      n263 = case shown="True" w598 {
        tunnel: w602 -> [_ w608]
        frame False {
        }
        frame True {
          n264 = call "Clipped_Hist_Check.vi"("Histogram Array"=w608) -> ()  [unwired: 1 out]
        }
      }
    }
    frame #14 {
      n265 = call "Multi_moments_LDA+_An.vi"("Timescales"=w610, "Measurement top level?"="Measurement top level?", "Vari Spaced"=w611) -> ("Max Measurement time up"=→"Max Measurement time up":bool, "File info"=w613:string[], "Vel stat display"=w614:string[][])  [unwired: 1 in]
      "Vel stat display" <- w614
      n266 = global write "Meas_global.vi" "Vel stats info for files"(w613) -> ()
      n267 = global write "Meas_global.vi" "Vel stat display"(w614) -> ()
    }
  }
